vi "YSCS_0-ADD8.vi"(1 "结束位置":u32, 2 "校验起始位":u32, 3 "输入字符串":string) -> (0 "输出字符串":string)   [LabVIEW 2015]
doc: "校验和，将从校验起始位开始到结束位置的数据累加求和，然后取负数"
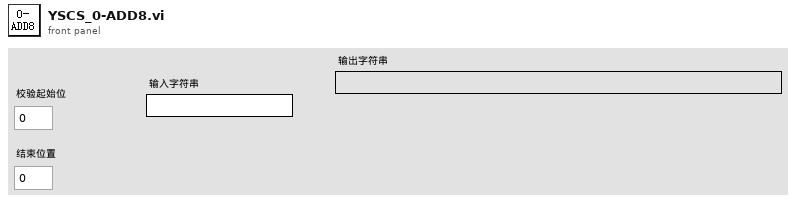
[diagram p1: front panel]
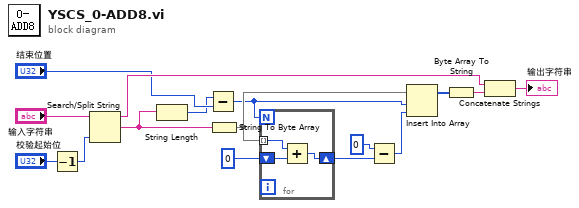
[diagram p0: block diagram]
diagram:
  n1 = Decrement(x="校验起始位") -> (x-1=w5:u32)
  n2 = Search/Split String(string="输入字符串", offset (0)=w5) -> (substring before match=w13:string, match + rest of string=w2:string)  [unwired: 1 in, 1 out]
  n3 = String Length(string=w2) -> (length=w1:i32)
  n4 = Subtract(x=w1, y="结束位置") -> (x-y=w3:u32)
  n5 = String To Byte Array(string=w2) -> (unsigned byte array=w10:u8[])
  n6 = for {
    N: w3 -> [_]
    tunnel: w10 -> [w17] mode=indexing
    shift-right: [w19] -> w14
    shift-left: u8 0 -> [w18]
    n7 = Add(x=w17, y=w18) -> (x+y=w19:u8)
  }
  n8 = Subtract(x=u8 0, y=w14) -> (x-y=w9:u8)
  n9 = Insert Into Array(array=w10, index=w3, new element=w9) -> (w8:u8[])
  n10 = Byte Array To String(unsigned byte array=w8) -> (string=w12:string)
  n11 = Concatenate Strings(w13, w12) -> (→"输出字符串":string)
